vi "初级计算器.vi"() -> ()   [LabVIEW 2018]
panel:
  in  "/":bool
  in  "*":bool
  in  "-":bool
  in  "+":bool
  out "结果":dbl format="%#_10g"
  in  "输入2":dbl
  in  "输入1":dbl
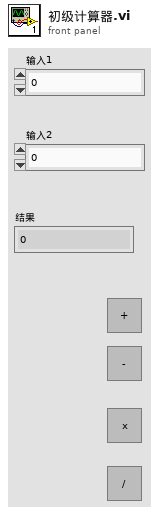
[diagram p1: front panel]
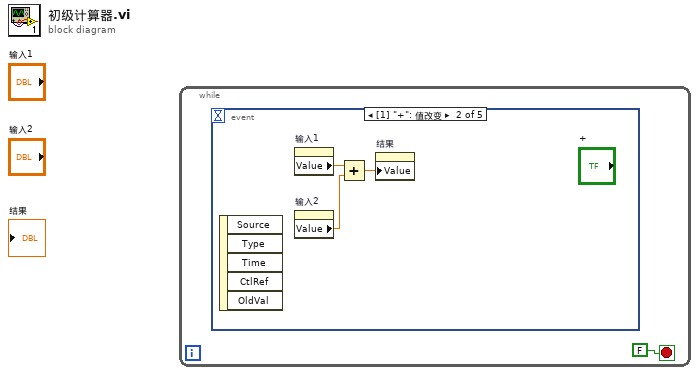
[diagram p0: block diagram]
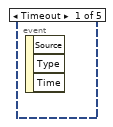
[diagram p2: hidden frame]
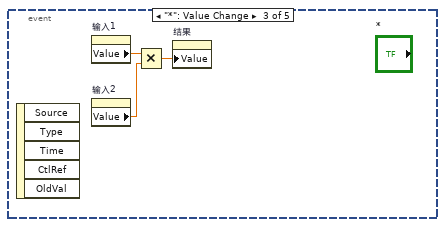
[diagram p3: hidden frame]
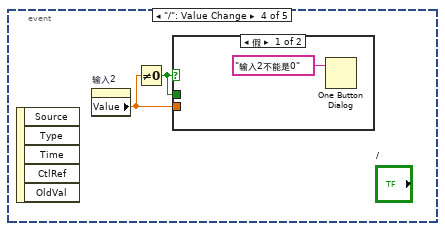
[diagram p4: hidden frame]
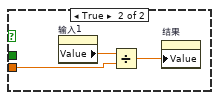
[diagram p5: hidden frame]
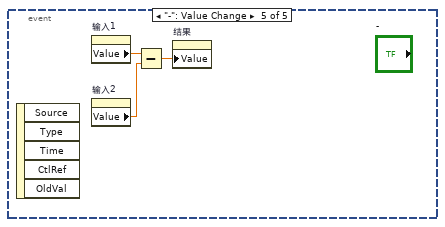
[diagram p6: hidden frame]
diagram:
  n1 = while {
    stop <- FALSE stop-if-true
    n2 = event shown="[1] \"+\": 值改变" {
      selector: _ -> [_ _ _ _ _]
      dyn-events: _ -> [_ _ _ _ _]
      timeout: _ -> [_ _ _ _ _]
      event Timeout {
        n3 = event-data() -> ()  [unwired: 1 in, 3 out]
      }
      event "+": Value Change {
        n4 = event-data() -> ()  [unwired: 1 in, 5 out]
        n5 = property on="输入1" class="DigNum (严格)"() -> ("Value"=w4:dbl)  [unwired: 2 in, 2 out]
        n6 = property on="输入2" class="DigNum (严格)"() -> ("Value"=w3:dbl)  [unwired: 2 in, 2 out]
        n7 = Add(x=w4, y=w3) -> (x+y=w2:dbl)
        n8 = property on="结果" class="DigNum (严格)"("Value"=w2) -> ()  [unwired: 2 in, 2 out]
      }
      event "*": Value Change {
        n9 = event-data() -> ()  [unwired: 1 in, 5 out]
        n10 = property on="输入1" class="DigNum (严格)"() -> ("Value"=w7:dbl)  [unwired: 2 in, 2 out]
        n11 = property on="输入2" class="DigNum (严格)"() -> ("Value"=w6:dbl)  [unwired: 2 in, 2 out]
        n12 = Multiply(x=w7, y=w6) -> (x*y=w5:dbl)
        n13 = property on="结果" class="DigNum (严格)"("Value"=w5) -> ()  [unwired: 2 in, 2 out]
      }
      event "/": Value Change {
        n14 = event-data() -> ()  [unwired: 1 in, 5 out]
        n15 = property on="输入2" class="DigNum (严格)"() -> ("Value"=w9:dbl)  [unwired: 2 in, 2 out]
        n16 = Not Equal To 0?(x=w9) -> (x != 0?=w8:bool)
        n17 = case shown="假" w8 {
          tunnel: w9 -> [_ w12]
          tunnel: w8 -> [_ _]
          frame False {
            n18 = One Button Dialog(message="输入2不能是0" ("消息")) -> ()  [unwired: 1 in, 1 out]
          }
          frame True {
            n19 = property on="输入1" class="DigNum (严格)"() -> ("Value"=w13:dbl)  [unwired: 2 in, 2 out]
            n20 = Divide(x=w13, y=w12) -> (x/y=w11:dbl)
            n21 = property on="结果" class="DigNum (严格)"("Value"=w11) -> ()  [unwired: 2 in, 2 out]
          }
        }
      }
      event "-": Value Change {
        n22 = event-data() -> ()  [unwired: 1 in, 5 out]
        n23 = property on="输入1" class="DigNum (严格)"() -> ("Value"=w16:dbl)  [unwired: 2 in, 2 out]
        n24 = property on="输入2" class="DigNum (严格)"() -> ("Value"=w15:dbl)  [unwired: 2 in, 2 out]
        n25 = Subtract(x=w16, y=w15) -> (x-y=w14:dbl)
        n26 = property on="结果" class="DigNum (严格)"("Value"=w14) -> ()  [unwired: 2 in, 2 out]
      }
    }
  }
